vi "Read Execution time.vi"(11 "Properties.Assert in":refnum<class "Properties.Assert.lvclass">) -> (2 "Execution time (s)":dbl=-1.0, 3 "Properties.Assert out":refnum<class "Properties.Assert.lvclass">)   [LabVIEW 2013, in "Caraya.lvlib" / "Properties.Assert.lvclass"]
uses:
  Properties.Assert.lvclass
  Properties.Assert.lvclass/Properties.Assert.ctl
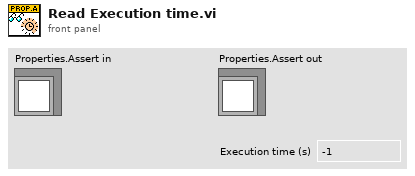
[diagram p1: front panel]
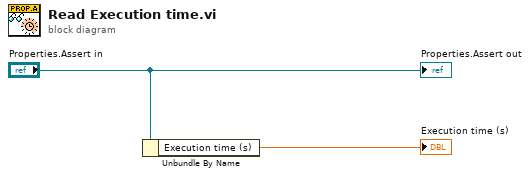
[diagram p0: block diagram]
diagram:
  n1 = Unbundle By Name("Properties.Assert in") -> ("Execution time (s)"=→"Execution time (s)":dbl)
  "Properties.Assert out" <- "Properties.Assert in"
